vi "XMLDataStructureUpdate.vi"(8 "error in (no error)":errorcluster, 9 "NewType In":T1 {"AllStepTypeData"."MoveData"."Mode" items=["Abs"=2, "Inc"=3]; "AllStepTypeData"."MoveData"."Axis" items=["X"=1, "Y"=2, "Z"=3, "Rotation"=4]}, 10 "XMLString In":string) -> (0 "error out":errorcluster, 1 "NewType Out":T1 {"AllStepTypeData"."MoveData"."Mode" items=["Abs"=2, "Inc"=3]; "AllStepTypeData"."MoveData"."Axis" items=["X"=1, "Y"=2, "Z"=3, "Rotation"=4]})   [LabVIEW 2014, in "Project.lvclass"]
uses:
  Project.lvclass
  StepSetupDataTypeDefine.ctl
  StepData/Control/AllStepTypeData.ctl
  StepData/Control/StepTypeEnum.ctl
  StepData/Control/MoveData.ctl
  StepData/Control/MeasureData.ctl
  StepData/StepData.lvclass
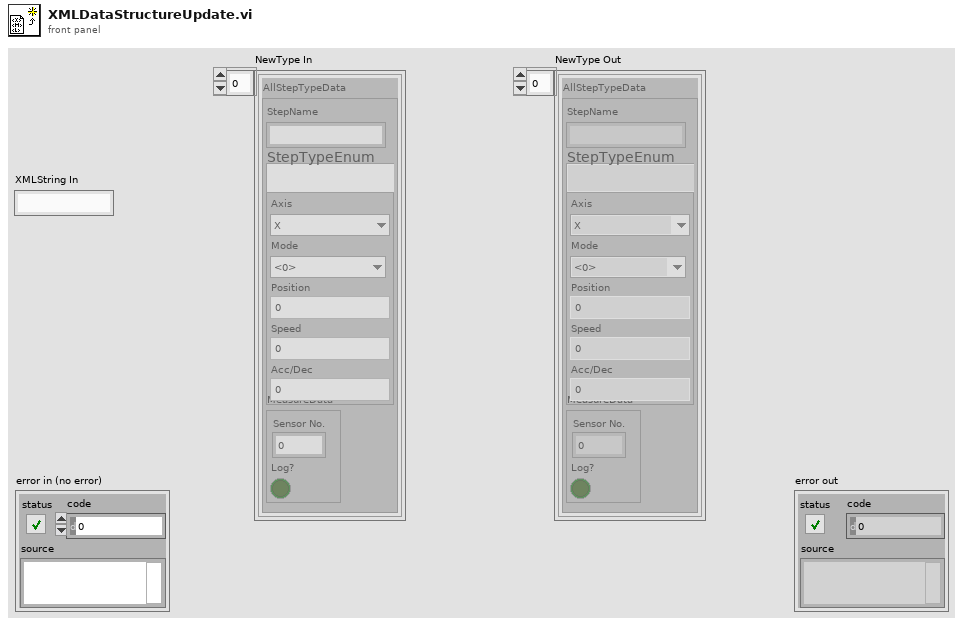
[diagram p1: front panel]
types:
  T1 = typedef "Project.lvclass/StepSetupDataTypeDefine.ctl" = cluster{"AllStepTypeData":T2}[]
  T2 = typedef "StepData.lvclass/AllStepTypeData.ctl" = cluster{"StepName":string, "StepTypeEnum":T3, "MoveData":T4, "MeasureData":T5}
  T3 = typedef "StepData.lvclass/StepTypeEnum.ctl" = enum16{"Move", "Measure"}
  T4 = typedef "StepData.lvclass/MoveData.ctl" = cluster{"Axis":u16, "Position":dbl, "Speed":dbl, "Acc/Dec":dbl, "Mode":u16}
  T5 = typedef "StepData.lvclass/MeasureData.ctl" = cluster{"Sensor No.":i32, "Log?":bool}
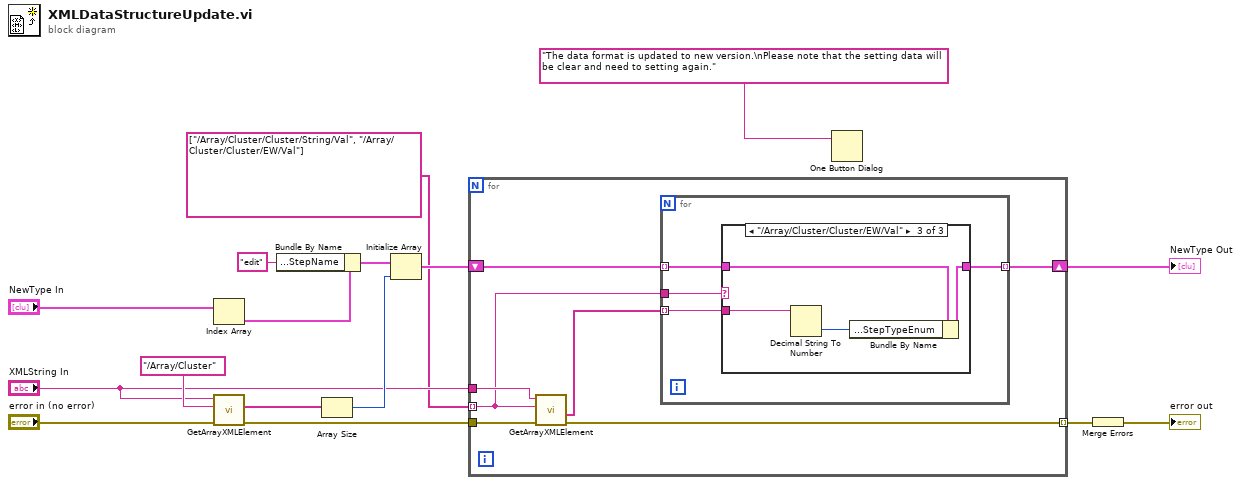
[diagram p0: block diagram]
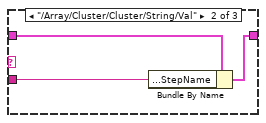
[diagram p3: hidden frame]
diagram:
  n1 = Index Array(array="NewType In") -> (element=w14:cluster{"AllStepTypeData":T2})  [unwired: 1 in]
  n2 = call "GetArrayXMLElement.vi"("error in (no error)"="error in (no error)", "XPathExpression"="/Array/Cluster", "XMLString"="XMLString In") -> ("error out"=w6:errorcluster, "XMLStringArray"=w9:string[])  [unwired: 6 in, 1 out]
  n3 = Bundle By Name(cluster=w14, "AllStepTypeData.StepName"="edit") -> (w12:cluster{"AllStepTypeData":T2})
  n4 = Array Size(array=w9) -> (size(s)=w8:i32)
  n5 = Initialize Array(w12, w8) -> (w5:cluster{"AllStepTypeData":T2}[])
  n6 = for {
    tunnel: "XMLString In" -> [w22]
    tunnel: w6 -> [w23]
    shift-right: [w18] -> w1
    shift-left: w5 -> [w19]
    tunnel: string[] ["/Array/Cluster/Cluster/String/Val", "/Array/Cluster/Cluster/EW/Val"] -> [w20] mode=indexing
    tunnel: [w17] -> w3 mode=indexing
    n7 = call "GetArrayXMLElement.vi"("error in (no error)"=w23, "XPathExpression"=w20, "XMLString"=w22) -> ("error out"=w17:errorcluster, "DataStringArrar"=w21:string[])  [unwired: 6 in, 1 out]
    n8 = for {
      tunnel: w21 -> [w26] mode=indexing
      tunnel: w20 -> [w27]
      tunnel: w19 -> [w25] mode=indexing
      tunnel: [w24] -> w18 mode=indexing
      n9 = case shown="\"/Array/Cluster/Cluster/EW/Val\"" w27 {
        tunnel: w26 -> [_ w29 w32]
        tunnel: w25 -> [w28 w31 w35]
        tunnel: [w28 w30 w34] -> w24
        frame Default {
        }
        frame "/Array/Cluster/Cluster/String/Val" {
          n10 = Bundle By Name(cluster=w31, "AllStepTypeData.StepName"=w29) -> (w30:cluster{"AllStepTypeData":T2})
        }
        frame "/Array/Cluster/Cluster/EW/Val" {
          n11 = Decimal String To Number(string=w32) -> (number=w33:i32)  [unwired: 2 in, 1 out]
          n12 = Bundle By Name(cluster=w35, "AllStepTypeData.StepTypeEnum"=w33) -> (w34:cluster{"AllStepTypeData":T2})
        }
      }
    }
  }
  "NewType Out" <- w1
  n13 = One Button Dialog(message="The data format is updated to new version.\nPlease note that the setting data will be clear and need to setting again.") -> ()  [unwired: 1 in, 1 out]
  n14 = Merge Errors(w3) -> (→"error out":errorcluster)
